vi "ULx Create Channel (CompI-Analog Input-Temperature).vi"(0 "task in":refnum<k24>, 5 "physical channels":refnum<k21>, 7 "units":i32(ring) items=["degC", "degF", "kelvin", "raw"], 11 "error in":errorcluster) -> (4 "task out":refnum<k24>, 15 "error out":errorcluster)   [LabVIEW 2020]
doc: "Creates channel(s) to measure temperature."
uses:
  C:/Users/William/Documents/LV 2020 builds/LeaktestDAQ/Source-v33/ULx_LV.dll
  ULx_LV.dll
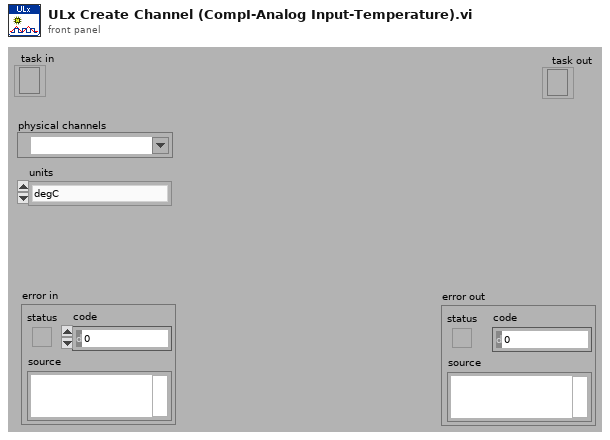
[diagram p1: front panel]
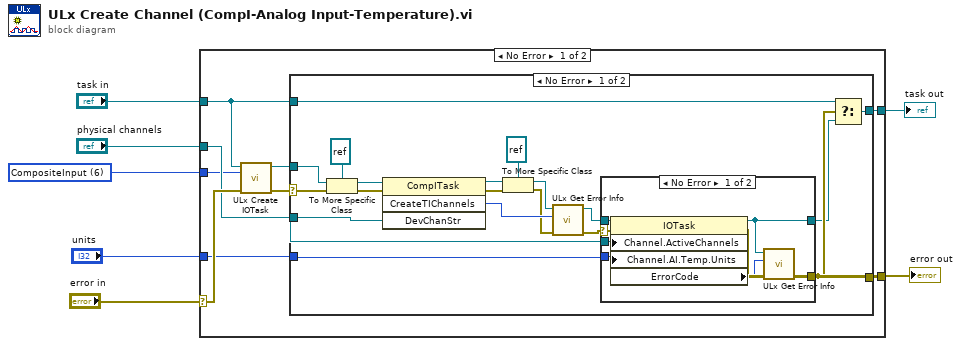
[diagram p0: block diagram]
diagram:
  w2 = 6 items=["AnalogInput", "AnalogOutput", "DigitalInput", "DigitalOutput", "CounterInput", "CounterOutput", "CompositeInput", "CompositeOutput", "TemperatureInput"] ("taskType")
  n1 = case shown="No Error" "error in" {
    selector: "error in" -> [w16 w48]
    tunnel: "task in" -> [w8 w47]
    tunnel: "physical channels" -> [w11 _]
    tunnel: [w14 w47] -> w5
    tunnel: [w13 w48] -> w4
    tunnel: w2 -> [w10 _]
    tunnel: "units" -> [w9 _]
    frame No Error {
      n2 = call "ULx Create IOTask.vi"("error in"=w16, "taskType"=w10, "i/o task in"=w8) -> ("error out"=w15:errorcluster, "i/o task out"=w12:refnum<k24>)  [unwired: 7 in]
      n3 = case shown="No Error" w15 {
        selector: w15 -> [w32 w46]
        tunnel: [w19 w46] -> w13
        tunnel: [w20 w45] -> w14
        tunnel: w12 -> [w30 _]
        tunnel: w11 -> [w26 _]
        tunnel: w9 -> [w27 _]
        tunnel: w8 -> [w17 w45]
        frame No Error {
          n4 = To More Specific Class(target class=refnum<k24> refnum, reference=w30, error in=w32) -> (specific class reference=w33:refnum<k24>, error out=w31:errorcluster)
          n5 = invoke class="CompITask" method="CreateTIChannels"(reference=w33, error in=w31, "DevChanStr"=w26) -> (reference out=w24:refnum<k24>, error out=w23:errorcluster, "CreateTIChannels"=w29:i32)  [unwired: 1 in, 1 out]
          n6 = To More Specific Class(target class=refnum<k24> refnum, reference=w24, error in=w23) -> (specific class reference=w21:refnum<k24>, error out=w22:errorcluster)
          n7 = call "ULx Get Error Info.vi"("error in"=w22, "ErrorCode"=w29, "task in"=w21) -> ("error out"=w28:errorcluster)  [unwired: 8 in]
          n8 = case shown="No Error" w28 {
            selector: w28 -> [w42 w44]
            tunnel: w21 -> [w41 w43]
            tunnel: w27 -> [w36 _]
            tunnel: w26 -> [w40 _]
            tunnel: [w37 w44] -> w19
            tunnel: [w35 w43] -> w18
            frame No Error {
              n9 = property class="IOTask"(reference=w41, error in=w42, "Channel.ActiveChannels"=w40, "Channel.AI.Temp.Units"=w36) -> (reference out=w35:refnum<k24>, error out=w38:errorcluster, "ErrorCode"=w39:i32)
              n10 = call "ULx Get Error Info.vi"("error in"=w38, "ErrorCode"=w39, "task in"=w35) -> ("error out"=w37:errorcluster)  [unwired: 8 in]
            }
            frame Error {
            }
          }
          n11 = Select(t=w17, s=w19, f=w18) -> (s? t:f=w20:refnum<k24>)
        }
        frame Error {
        }
      }
    }
    frame Error {
    }
  }
  "error out" <- w4
  "task out" <- w5
